vi "CaseStructure - Case Name to Group Name.vi"(11 "element":string) -> (3 "String":string)   [LabVIEW 2017, in "CSM-Helper.lvclass"]
uses:
  CSM-Helper.lvclass
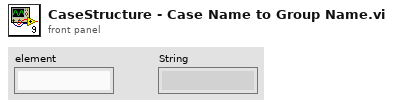
[diagram p1: front panel]
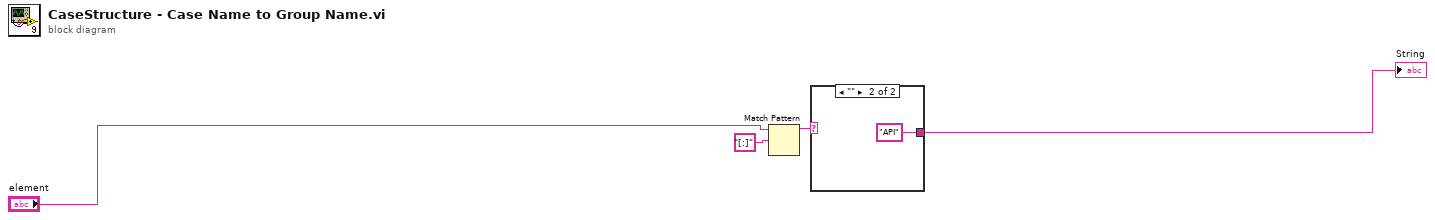
[diagram p0: block diagram]
diagram:
  n1 = Match Pattern(string="element", regular expression="[:]") -> (before substring=w1:string)  [unwired: 1 in, 3 out]
  n2 = case shown="\"\"" w1 {
    selector: w1 -> [w5 _]
    tunnel: [w5 "API"] -> w3
    frame "False", Default {
    }
    frame "" {
    }
  }
  "String" <- w3
